vi "Close Input Ref.vi"(8 "error in (no error)":errorcluster, 11 "AIT 429 in":refnum<class "AIT 429.lvclass">) -> (0 "error out":errorcluster, 3 "AIT 429 out":refnum<class "AIT 429.lvclass">)   [LabVIEW 2021, in "ARINC.lvlib" / "AIT 429.lvclass"]
uses:
  AIT 429.lvclass
  Abstract/Abstract.lvclass
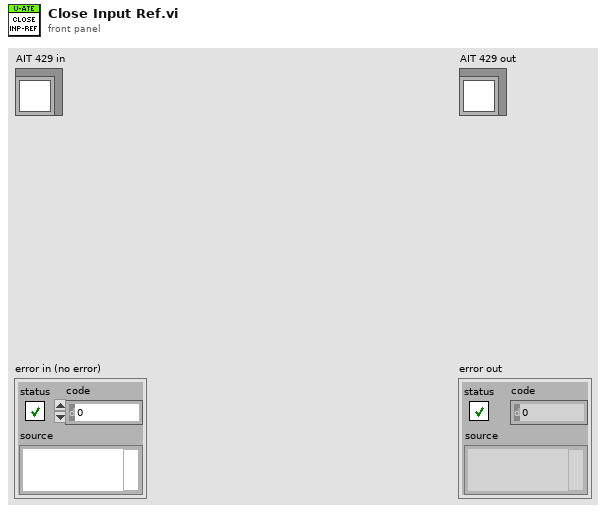
[diagram p1: front panel]
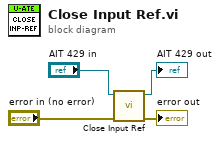
[diagram p0: block diagram]
diagram:
  n1 = call-parent "Close Input Ref.vi"("error in (no error)"="error in (no error)", "Abstract in"="AIT 429 in") -> ("error out"=→"error out":errorcluster, "Abstract out"=→"AIT 429 out":refnum<class "AIT 429.lvclass">)  [unwired: 8 in]
